vi "Create New Packed Library.vi"(8 "error in (no error)":errorcluster, 10 "Build specification name":string, 11 "Project Refnum":refnum<vi>) -> (0 "error out":errorcluster, 3 "PPL out":refnum<class "NI_AB_API_PPL.lvclass">)   [LabVIEW 2020, in "NI_AB_API_PPL.lvclass"]
uses:
  <vilib>/AppBuilder/AB_API/PPL/NI_AB_API_PPL.lvclass
  e:/builds/penguin/labview/branches/2020/dev/dist/vi.lib/AppBuilder/AB_API/Build/NI_AB_API_Build.lvclass
  <vilib>/AppBuilder/AB_Classes/PackedLib/AB_PackedLibrary.lvclass
  e:/builds/penguin/labview/branches/2020/dev/dist/vi.lib/AppBuilder/AB_Classes/Build/AB_Build.lvclass
  <vilib>/AppBuilder/AB_API/common/AB_API Build Object Type.ctl
  <vilib>/AppBuilder/AB_API/Build/NI_AB_API_Build.lvclass
panel:
  in  "TargetItem Refnum":refnum<vi>
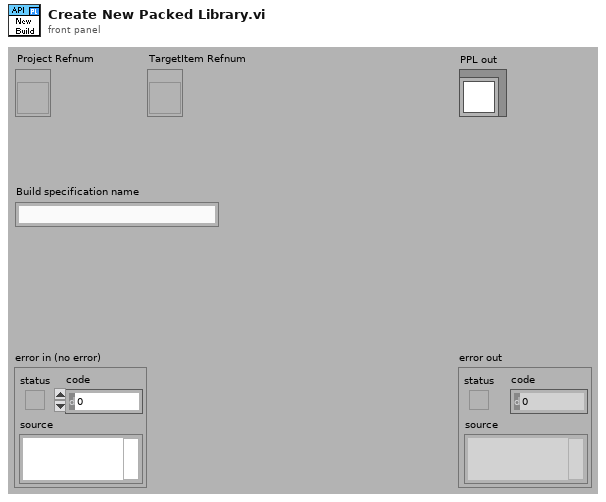
[diagram p1: front panel]
types:
  T1 = typedef "AB_API Build Object Type.ctl" = enum16{"Source Distribution", "DLL", "EXE", "Installer", "Zip File", "RESTful WS", "RTEXE", "Packed Library", "C Generation ", ".NET Interop Assembly"}
  T2 = typedef "ItemRef.ctl" = u64
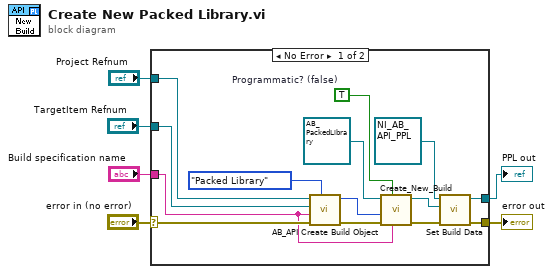
[diagram p0: block diagram]
diagram:
  n1 = case shown="No Error" "error in (no error)" {
    selector: "error in (no error)" -> [w17 w21]
    tunnel: [w10 w21] -> w5
    tunnel: [w9 _] -> w4
    tunnel: "Build specification name" -> [w16 _]
    tunnel: "Project Refnum" -> [w15 _]
    tunnel: "TargetItem Refnum" -> [w14 _]
    frame No Error {
      w13 = TRUE  # Programmatic? (false)
      n2 = call <vilib>:"AB_API Create Build Object.vi"("Build object type"=AB_API_Build_Object_Type."Packed Library", "error in (no error)"=w17, "Build spec name"=w16, "TargetItem Refnum"=w14, "Project Refnum"=w15) -> ("error out"=w20:errorcluster, "Build object"=w19:T2)  [unwired: 5 in]
      n3 = call-dynamic "Create_New_Build.vi"("buildSpecName"=w16, "Programmatic? (false)"=w13, "error in (no error)"=w20, "buildObject"=w19, "AB_PackedLibrary in"=refnum<class "AB_PackedLibrary.lvclass"> refnum ("AB_PackedLibrary.lvclass")) -> ("error out"=w11:errorcluster, "AB_PackedLibrary out"=w7:refnum<class "AB_PackedLibrary.lvclass">)  [unwired: 5 in]
      n4 = call <vilib>:"Set Build Data.vi"("error in (no error)"=w11, "AB_Build.lvclass"=w7, "NI_AB_API_Build in"=refnum<class "NI_AB_API_PPL.lvclass"> refnum ("AB_API_DLL.lvclass")) -> ("error out"=w10:errorcluster, "NI_AB_API_Build out"=w9:refnum<class "NI_AB_API_PPL.lvclass">)  [unwired: 7 in]
    }
    frame Error {
    }
  }
  "error out" <- w5
  "PPL out" <- w4
